vi "DantecHwInputScale.vi"(9 "Wind Speed Offset (m/s)":dbl, 10 "Wind Speed Scale ((m/s)/V^#)":dbl[](array[numeric]), 11 "Raw (V)":dbl) -> (3 "Wind Speed (m_s)":dbl)   [LabVIEW 2018]
uses:
  <vilib>/express/express arith-compare/Formula/XNode/ExpressFormulaBlockNode.xnode
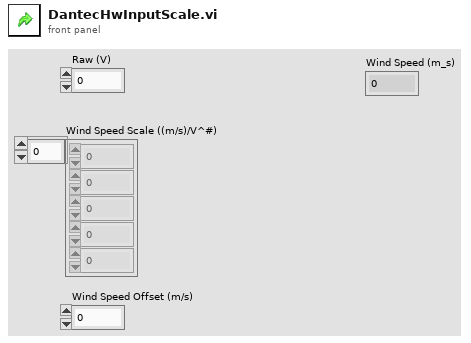
[diagram p1: front panel]
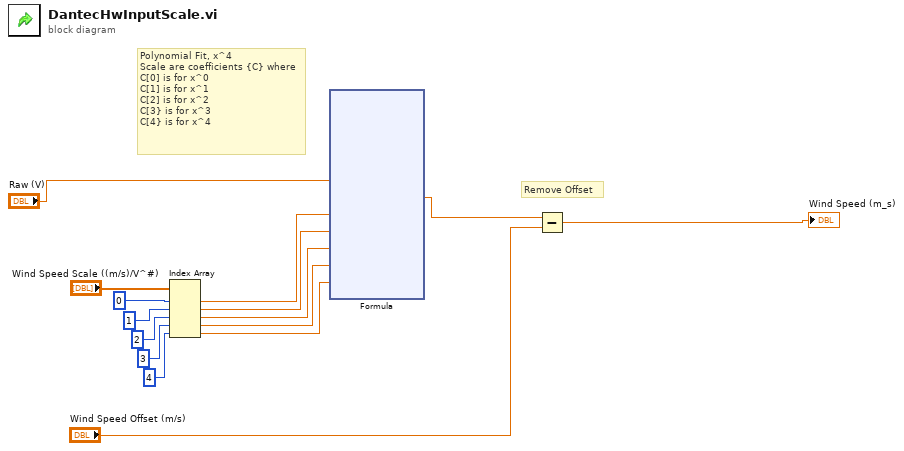
[diagram p0: block diagram]
diagram:
  # "Polynomial Fit, x^4\nScale are coefficients {C} where\nC[0] is for x^0\nC[1] is for x^1\nC[2] is for x^2\nC[3} is for x^3\nC[4} is for x^4"
  # "Remove Offset"
  n1 = Index Array(array="Wind Speed Scale ((m/s)/V^#)", index #1=0 ("index"), index #2=1 ("index"), index #3=2 ("index"), index #4=3 ("index"), index #5=4 ("index")) -> (element #1=w7:dbl, element #2=w6:dbl, element #3=w5:dbl, element #4=w4:dbl, element #5=w2:dbl)
  n2 = xnode "Formula"("X"="Raw (V)", "C0"=w7, "C1"=w6, "C2"=w5, "C3"=w4, "C4"=w2) -> ("Result"=w13:dbl)  [unwired: 1 in, 1 out]
  n3 = Subtract(x=w13, y="Wind Speed Offset (m/s)") -> (x-y=→"Wind Speed (m_s)":dbl)
